vi "Detection Logic to FPGA.vi"() -> ()   [LabVIEW 2026]
uses:
  <vilib>/rvi/Emulation/niFpgaGetClockAttributes.vi
  <vilib>/rvi/Emulation/niFpgaSctlEmulationGetInTimedLoop.vi
  <vilib>/rvi/Emulation/niFpgaEmulationReportErrorSimple.vi
  <extravilib>/ChannelInstances/Tag-bool/Instantiate.vi
  <vilib>/rvi/Emulation/niFpgaProcessEmulError.vi
  <vilib>/rvi/Emulation/niFpgaCriticalErrorInLSC.vi
  <vilib>/rvi/eio/common/nirviEmuTemplateMethod_errors.vi
  <vilib>/eio/EIONode/EIONode.xnode
  <extravilib>/ChannelInstances/Tag-bool.lvlib
panel:
  out "Last speed":u64
  out "Multiplier":u16
  in  "Random Number Max":u8=16
  out "Random Number":u8
  out "Score":u16
  in  "Speed Threshold, ticks":u64=3000
  out "Pressed":bool[](array[boolean])
  out "Valid":bool[](array[boolean])
  in  "Debounce Threshold, ticks":u64=1000
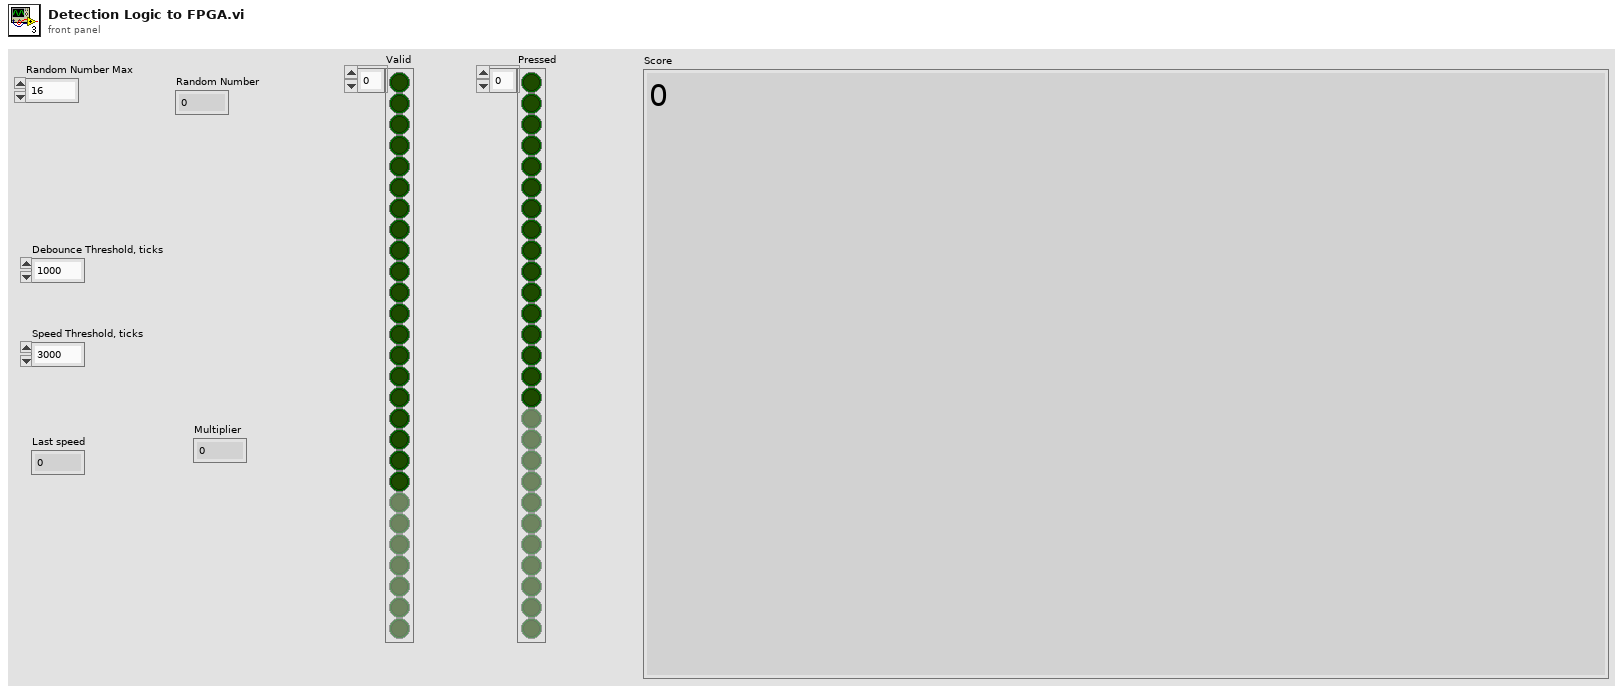
[diagram p1: front panel]
types:
  T1 = typedef "Tag-bool.lvlib/))Channel.ctl" = refnum<queue>
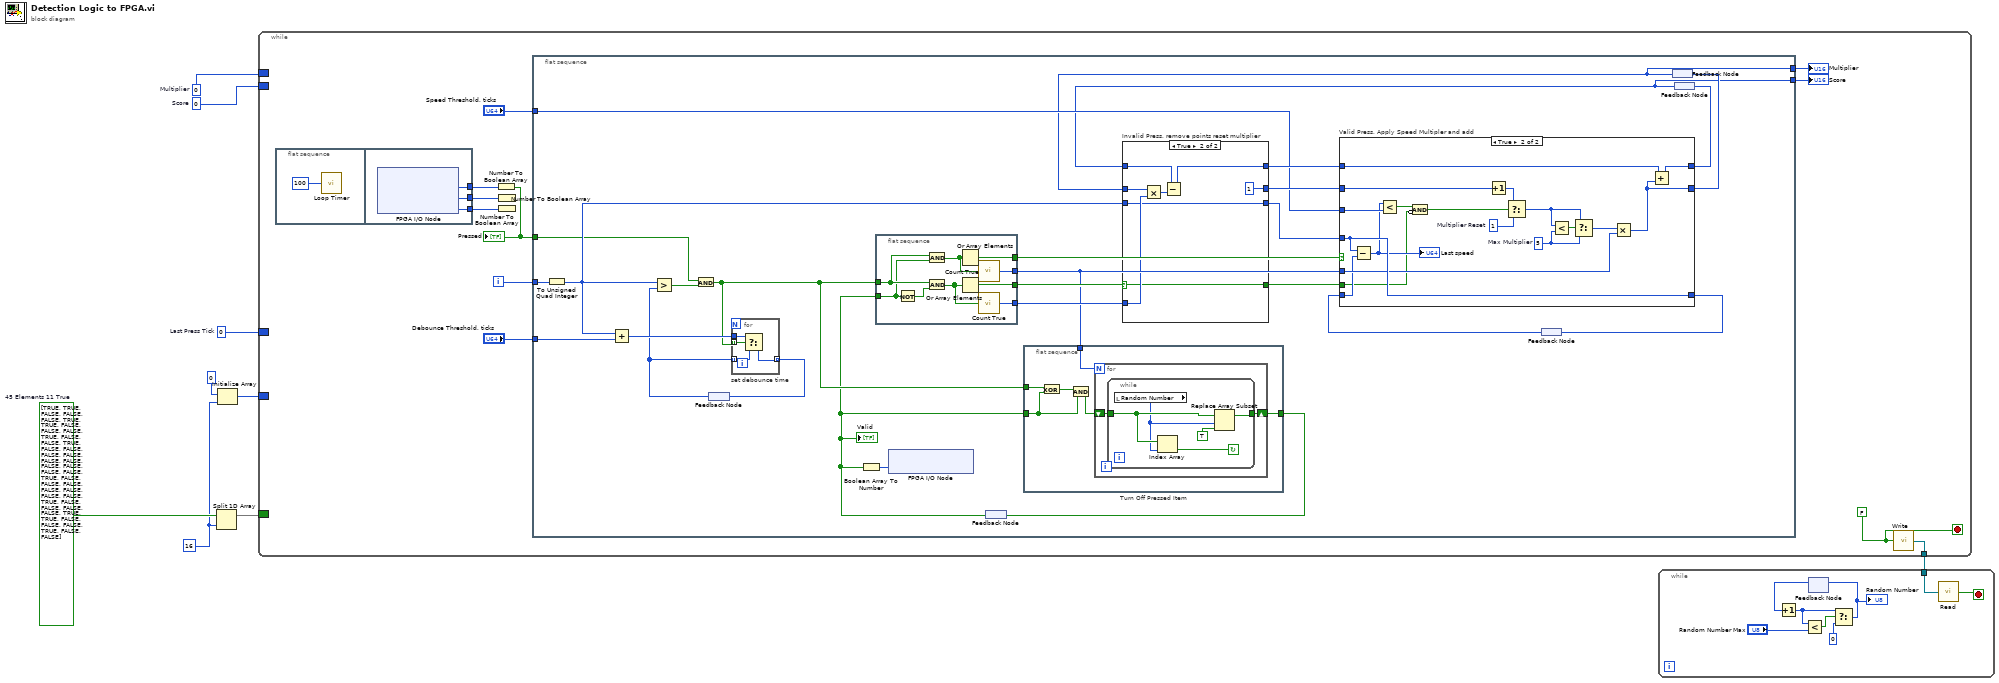
[diagram p0: block diagram]
diagram:
  w1 = u64 0  # Last Press Tick
  w2 = 16 ("index")
  w4 = bool[] [TRUE, TRUE, FALSE, FALSE, FALSE, TRUE, TRUE, FALSE, FALSE, FALSE, TRUE, FALSE, FALSE, TRUE, FALSE, FALSE, FALSE, FALSE, FALSE, FALSE, FALSE, FALSE, FALSE, FALSE, TRUE, FALSE, FALSE, FALSE, FALSE, FALSE, FALSE, FALSE, TRUE, FALSE, FALSE, FALSE, FALSE, TRUE, TRUE, FALSE, FALSE, FALSE, TRUE, FALSE, FALSE]  # 45 Elements 11 True
  w7 = u16 0  # Multiplier
  w6 = u16 0  # Score
  n1 = Split 1D Array(array=w4, index=w2) -> (first subarray=w3:bool[])  [unwired: 1 out]
  n2 = Initialize Array(u64 0 ("Bonus Threshold"), w2) -> (w8:u64[])
  n3 = while {
    border: w8 -> [_]
    border: w3 -> [_]
    border: w6 -> [_]
    border: w7 -> [_]
    tunnel: [w17] -> w5
    border: w1 -> [_]
    i -> [w20]
    stop <- w14 stop-if-true
    w14 = FALSE
    n4 = flat-sequence {
      tunnel: [w24] -> w13
      tunnel: [w23] -> w12
      tunnel: [w22] -> w11
      frame #0 {
        n5 = call "Loop Timer"("Count(uSec)"=u32 100) -> ()  [unwired: 1 out]
      }
      frame #1 {
        n6 = xnode "FPGA I/O Node"() -> ("Bank-01/DI15:0"=w24:u16, "Bank-02/DI15:0"=w23:u16, "Bank-03/DI15:0"=w22:u16)  [unwired: 3 in, 3 out]
      }
    }
    n7 = Number To Boolean Array(number=w13) -> (Boolean array=w15:bool[])
    "Pressed" <- w15
    n8 = Number To Boolean Array(number=w12) -> ()  [unwired: 1 out]
    n9 = Number To Boolean Array(number=w11) -> ()  [unwired: 1 out]
    n10 = flat-sequence {
      tunnel: w20 -> [w50]
      tunnel: "Debounce Threshold, ticks" -> [w48]
      tunnel: "Speed Threshold, ticks" -> [w40]
      tunnel: w15 -> [w36]
      tunnel: [w27] -> w16
      tunnel: [w28] -> w10
      frame #0 {
        n11 = To Unsigned Quad Integer(1:w50) -> (0:w39:u64)
        n12 = Add(x=w39, y=w48) -> (x+y=w49:u64)
        n13 = feedback #1() -> (w45:u64[])
        n14 = Greater?(x=w39, y=w45) -> (0:w51:bool[])
        n15 = And(x=w36, y=w51) -> (x .and. y?=w34:bool[])
        n16 = for "set debounce time" {
          tunnel: w34 -> [w101] mode=indexing
          tunnel: w45 -> [w99] mode=indexing
          tunnel: w49 -> [w100]
          tunnel: [w98] -> w46 mode=indexing
          n17 = Select(t=w100, s=w101, f=w99) -> (s? t:f=w98:u64)
        }
        n18 = feedback-in #1(w46) -> ()
        n19 = flat-sequence {
          tunnel: w34 -> [w110]
          tunnel: [w108] -> w44
          tunnel: w29 -> [w107]
          tunnel: [w106] -> w47
          tunnel: [w102] -> w43
          tunnel: [w104] -> w35
          frame #0 {
            n20 = Not(x=w107) -> (.not. x?=w109:bool[])
            n21 = And(x=w110, y=w107) -> (x .and. y?=w105:bool[])
            n22 = And(x=w110, y=w109) -> (x .and. y?=w103:bool[])
            n23 = Or Array Elements(Boolean array=w105) -> (logical OR=w106:bool)
            n24 = Or Array Elements(Boolean array=w103) -> (logical OR=w108:bool)
            n25 = call "Count True.vi"("Booleans"=w105) -> ("Count"=w104:u16)  [unwired: 14 in]
            n26 = call "Count True.vi"("Booleans"=w103) -> ("Count"=w102:u16)  [unwired: 14 in]
          }
        }
        n27 = feedback #2() -> (w29:bool[])
        "Valid" <- w29
        n28 = Boolean Array To Number(Boolean array=w29) -> (number=w30:u32)
        n29 = xnode "FPGA I/O Node"("Bank-01/DO15:0"=w30) -> ()  [unwired: 1 in, 1 out]
        n30 = feedback-in #2(w32) -> ()
        n31 = flat-sequence "Turn Off Pressed Item" {
          tunnel: w34 -> [w55]
          tunnel: [w54] -> w32
          tunnel: w29 -> [w56]
          tunnel: w35 -> [w52]
          frame #0 {
            n32 = Exclusive Or(1:w56, 2:w55) -> (0:w57:bool[])
            n33 = And(x=w57, y=w56) -> (x .and. y?=w53:bool[])
            n34 = for {
              N: w52 -> [_]
              shift-right: [w58] -> w54
              shift-left: w53 -> [w59]
              n35 = while {
                tunnel: w59 -> [w63]
                tunnel: [w62] -> w58
                stop <- w64 continue-if-true
                n36 = local read "Random Number"() -> (w61:u8)
                n37 = Index Array(array=w63, index=w61) -> (element=w64:bool)
                n38 = Replace Array Subset(array=w63, new element=TRUE ("new element/subarray"), index=w61) -> (w62:bool[])
              }
            }
          }
        }
        n39 = feedback #3() -> (w26:u64)
        n40 = feedback #4() -> (w27:u16)
        n41 = feedback #5() -> (w28:u16)
        n42 = case "Invalid Press, remove points reset multiplier" shown="True" w44 {
          selector: w44 -> [w65 w71]
          tunnel: w27 -> [w68 w74]
          tunnel: w39 -> [w66 w69]
          tunnel: [w68 u16 1 ("Multiplier")] -> w41
          tunnel: w28 -> [w67 w75]
          tunnel: [w67 w76] -> w42
          tunnel: w43 -> [_ w73]
          tunnel: [w66 w69] -> w38
          tunnel: [w65 w71] -> w25
          frame False {
          }
          frame True {
            n43 = Multiply(x=w74, y=w73) -> (x*y=w72:u16)
            n44 = Subtract(x=w75, y=w72) -> (x-y=w76:u16)
          }
        }
        n45 = case "Valid Press, Apply Speed Multipler and add" shown="True" w47 {
          tunnel: w42 -> [w78 w96]
          tunnel: w41 -> [w79 w93]
          tunnel: [w79 w86] -> w31
          tunnel: [w78 w97] -> w33
          tunnel: w40 -> [_ w95]
          tunnel: [w77 w92] -> w37
          tunnel: w38 -> [_ w92]
          tunnel: w35 -> [_ w87]
          tunnel: w26 -> [w77 w82]
          tunnel: w25 -> [_ w80]
          frame False {
          }
          frame True {
            w90 = u16 5  # Max Multiplier
            w88 = u16 1  # Multiplier Reset
            n46 = Subtract(x=w92, y=w82) -> (x-y=w85:u64)
            "Last speed" <- w85
            n47 = Less?(x=w85, y=w95) -> (x < y?=w94:bool)
            n48 = Compound Arithmetic op=AND(w94, invert w80) -> (w81:bool)
            n49 = Increment(x=w93) -> (x+1=w89:u16)
            n50 = Select(t=w89, s=w81, f=w88) -> (s? t:f=w83:u16)
            n51 = Less?(x=w83, y=w90) -> (x < y?=w91:bool)
            n52 = Select(t=w83, s=w91, f=w90) -> (s? t:f=w84:u16)
            n53 = Multiply(x=w84, y=w87) -> (x*y=w86:u16)
            n54 = Add(x=w96, y=w86) -> (x+y=w97:u16)
          }
        }
        n55 = feedback-in #3(w37) -> ()
        n56 = feedback-in #4(w31) -> ()
        n57 = feedback-in #5(w33) -> ()
      }
    }
    n58 = call <extravilib>:"Write.vi"("element"=w14) -> ("channel"=w17:T1)  [unwired: 1 out]
    "Score" <- w10
    "Multiplier" <- w16
  }
  n59 = while {
    tunnel: w5 -> [w113]
    stop <- w112 stop-if-true
    n60 = feedback #6() -> (w115:u8)  [unwired: 1 in]
    n61 = Increment(x=w115) -> (x+1=w111:u8)
    n62 = Less?(x=w111, y="Random Number Max") -> (x < y?=w116:bool)
    n63 = Select(t=w111, s=w116, f=u8 0) -> (s? t:f=w118:u8)
    "Random Number" <- w118
    n64 = feedback-in #6(w118) -> ()
    n65 = call <extravilib>:"Read.vi"("channel"=w113) -> ("element"=w112:bool)  [unwired: 1 in, 1 out]
  }
